vi "Read ConvBox Handler.vi"(8 "error in (no error)":errorcluster, 11 "Listener in":refnum<class "Listener.lvclass">) -> (0 "error out":errorcluster, 3 "Listener out":refnum<class "Listener.lvclass">)   [LabVIEW 2019, in "Listener.lvclass"]
uses:
  Listener.lvclass
  Listener.lvclass/Listener.ctl
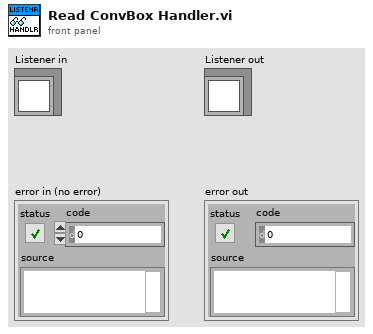
[diagram p1: front panel]
types:
  T1 = typedef "Listener.lvclass/RS-xxx To GPIB ConvBox Data Structure.ctl" = cluster{"Data":string, "Command Messages Read":string[], "Address":string}
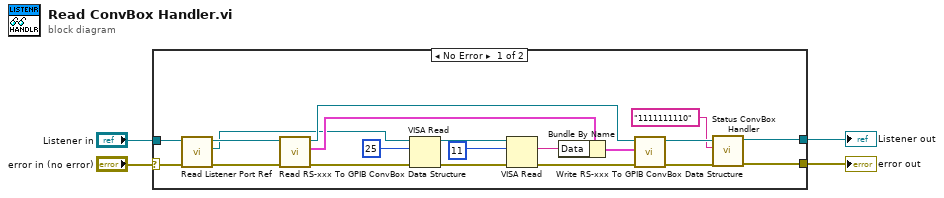
[diagram p0: block diagram]
diagram:
  n1 = case shown="No Error" "error in (no error)" {
    selector: "error in (no error)" -> [w8 w25]
    tunnel: "Listener in" -> [w9 w26]
    tunnel: [w12 w25] -> w2
    tunnel: [w11 w26] -> w1
    frame No Error {
      n2 = call "Read Listener Port Ref.vi"("error in (no error)"=w8, "Listener in"=w9) -> ("error out"=w6:errorcluster, "Listener Port Ref"=w5:refnum<visa-resource-name>, "Listener out"=w7:refnum<class "Listener.lvclass">)  [unwired: 7 in]
      n3 = call-dynamic "Read RS-xxx To GPIB ConvBox Data Structure.vi"("error in (no error)"=w6, "Listener in"=w7) -> ("error out"=w10:errorcluster, "RS-xxx To GPIB ConvBox Data Structure"=w20:T1, "Listener out"=w15:refnum<class "Listener.lvclass">)  [unwired: 7 in]
      n4 = VISA Read(VISA resource name=w5, byte count=u32 25, error in (no error)=w10) -> (VISA resource name out=w23:refnum<visa-resource-name>, error out=w22:errorcluster)  [unwired: 2 out]
      n5 = VISA Read(VISA resource name=w23, byte count=u32 11, error in (no error)=w22) -> (read buffer=w19:string, error out=w18:errorcluster)  [unwired: 2 out]
      n6 = Bundle By Name(cluster=w20, "Data"=w19) -> (w16:T1)
      n7 = call-dynamic "Write RS-xxx To GPIB ConvBox Data Structure.vi"("error in (no error)"=w18, "RS-xxx To GPIB ConvBox Data Structure"=w16, "Listener in"=w15) -> ("error out"=w17:errorcluster, "Listener out"=w14:refnum<class "Listener.lvclass">)  [unwired: 7 in]
      n8 = call "Status ConvBox Handler.vi"("error in(no error)"=w17, "Value In"="1111111110" ("write buffer"), "Listener in"=w14) -> ("error out"=w12:errorcluster, "Listener out"=w11:refnum<class "Listener.lvclass">)  [unwired: 7 in]
    }
    frame Error {
    }
  }
  "error out" <- w2
  "Listener out" <- w1
